vi "Linear Intopolation.vi"(0 "x1":dbl format="%0.2f", 1 "x2":dbl format="%0.2f", 2 "y1":dbl format="%0.2f", 3 "y2":dbl format="%0.2f", 4 "x":dbl format="%0.2f") -> (5 "y":dbl format="%0.2f")   [LabVIEW 2017, in "NI_PtbyPt.lvlib"]
uses:
  <vilib>/ptbypt/NI_PtbyPt.lvlib
panel:
  # "Linear interpolation"
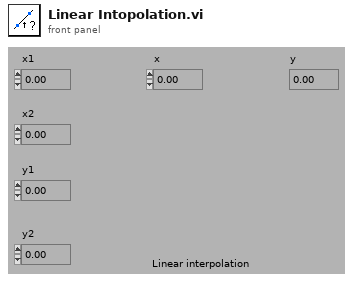
[diagram p1: front panel]
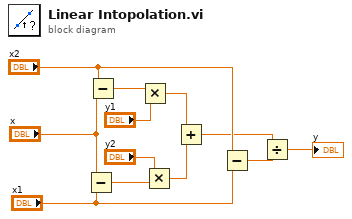
[diagram p0: block diagram]
diagram:
  n1 = Subtract(x="x", y="x1") -> (x-y=w8:dbl)
  n2 = Subtract(x="x2", y="x") -> (x-y=w9:dbl)
  n3 = Multiply(x=w9, y="y1") -> (x*y=w7:dbl)
  n4 = Multiply(x="y2", y=w8) -> (x*y=w6:dbl)
  n5 = Add(x=w7, y=w6) -> (x+y=w5:dbl)
  n6 = Subtract(x="x2", y="x1") -> (x-y=w4:dbl)
  n7 = Divide(x=w5, y=w4) -> (x/y=→"y":dbl)
